vi "main_subVi.vi"() -> ()   [LabVIEW 2020]
panel:
  in  "Enum":enum16{"add", "sub", "mul", "div"}(ring)
  out "C":dbl
  in  "B":dbl
  in  "A":dbl
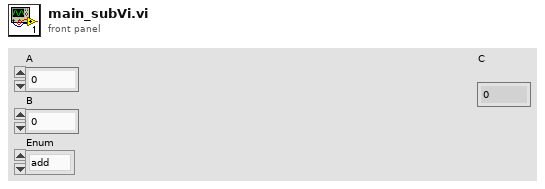
[diagram p1: front panel]
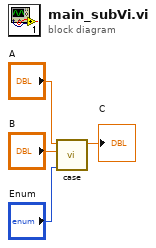
[diagram p0: block diagram]
diagram:
  n1 = call "case.vi"("Enum"="Enum", "B"="B", "A"="A") -> ("C"=→"C":dbl)  [unwired: 8 in]
